vi "lcmtestyest.vi"() -> ()   [LabVIEW 2015]
uses:
  rio_Global.vi
panel:
  out "error out 2":errorcluster
  in  "time-to-live (1)":u16=1
  in  "error in (no error)":errorcluster
  in  "port":u16
  out "error out":errorcluster
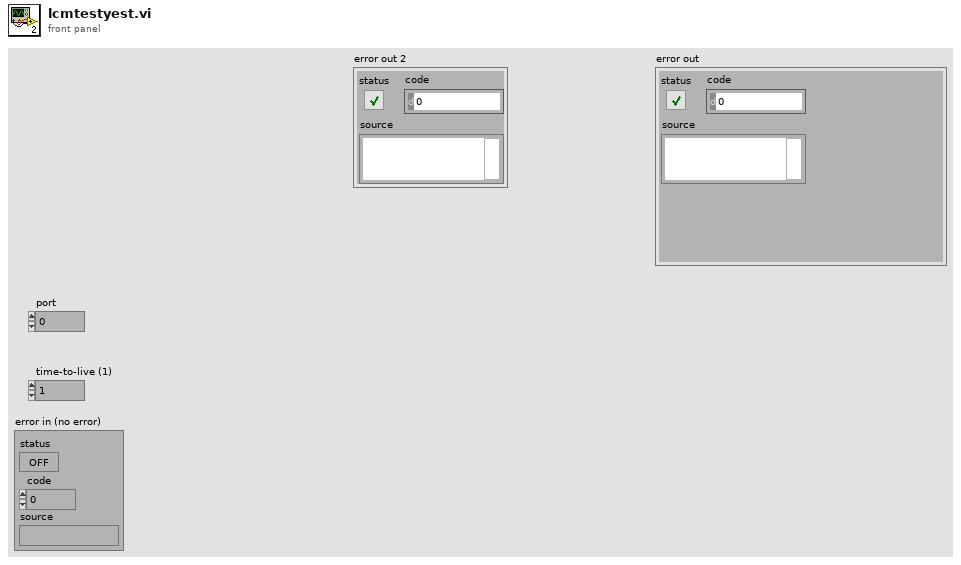
[diagram p1: front panel]
types:
  T1 = cluster{"connection ID":refnum<k16>, "net address":u32, "port":u16}
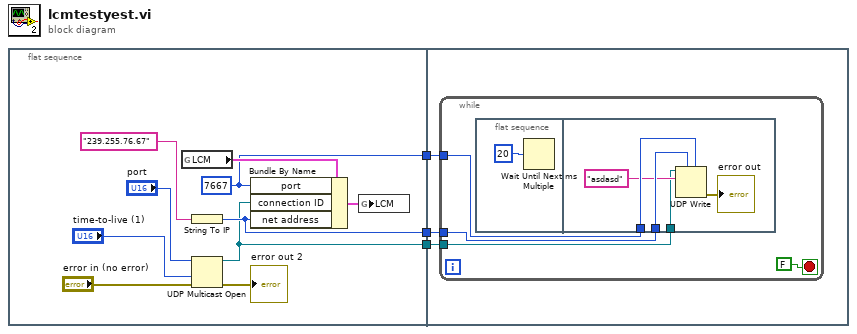
[diagram p0: block diagram]
diagram:
  n1 = flat-sequence {
    tunnel: [w6] -> w3
    tunnel: [w10] -> w2
    tunnel: [w5] -> w1
    tunnel: w3 -> [w16]
    tunnel: w2 -> [w15]
    tunnel: w1 -> [w14]
    frame #0 {
      w10 = u16 7667 ("port")
      n2 = global read "rio_Global.vi" "LCM"() -> (w13:T1)
      n3 = String To IP(1:"239.255.76.67" ("name")) -> (0:w6:u32)
      n4 = UDP Multicast Open(8:"error in (no error)", 9:"time-to-live (1)", 11:"port") -> (0:→"error out 2":errorcluster, 3:w5:refnum<k16>)  [unwired: 1 in, 2 out]
      n5 = Bundle By Name(cluster=w13, "port"=w10, "connection ID"=w5, "net address"=w6) -> (w12:T1)
      n6 = global write "rio_Global.vi" "LCM"(w12) -> ()
    }
    frame #1 {
      n7 = while {
        tunnel: w16 -> [w19]
        tunnel: w15 -> [w18]
        tunnel: w14 -> [w17]
        stop <- FALSE stop-if-true
        n8 = flat-sequence {
          tunnel: w19 -> [w26]
          tunnel: w18 -> [w25]
          tunnel: w17 -> [w22]
          frame #0 {
            n9 = Wait Until Next ms Multiple(millisecond multiple=u32 20) -> ()  [unwired: 1 out]
          }
          frame #1 {
            n10 = UDP Write(address=w26, port or service name=w25, connection ID=w22, data in="asdasd") -> (error out=→"error out":errorcluster)  [unwired: 2 in, 1 out]
          }
        }
      }
    }
  }
